vi "ROI-databuffer.vi"(4 "array in":cluster{"x":sgl, "y":sgl}[](array[cluster]), 5 "command":enum16{"get", "set", "clear", "append"}(ring)) -> (1 "array out":cluster{"x":sgl, "y":sgl}[](array[cluster]))   [LabVIEW 2015]
panel:
  in  "point in":cluster{"x":sgl, "y":sgl}
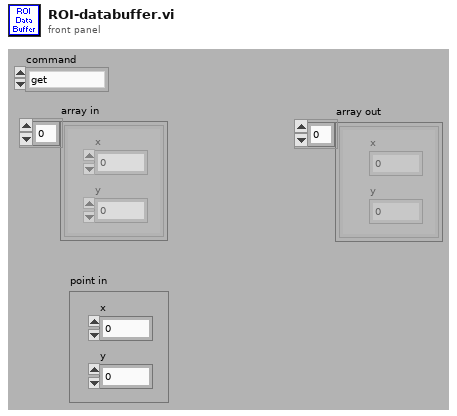
[diagram p1: front panel]
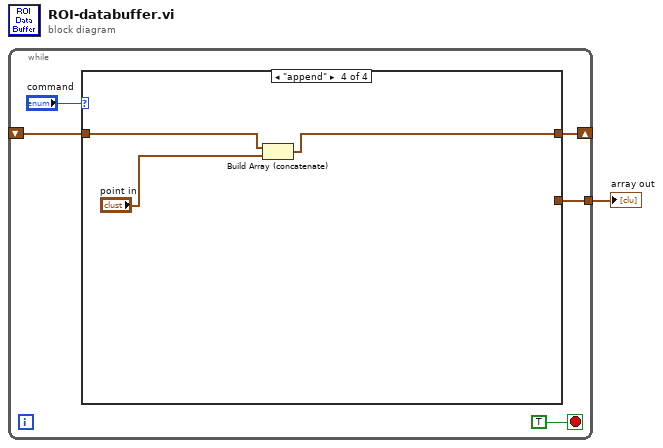
[diagram p0: block diagram]
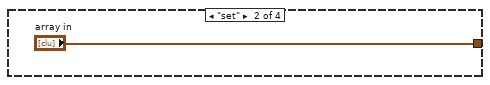
[diagram p3: hidden frame]
diagram:
  n1 = while {
    shift-right: [w4] -> _
    shift-left: _ -> [w5]
    tunnel: [w3] -> w1
    stop <- TRUE stop-if-true
    n2 = case shown="\"append\"" "command" {
      tunnel: [w7 "array in" _ w11] -> w4
      tunnel: w5 -> [w7 _ _ w10]
      tunnel: [w7 _ _ _] -> w3
      frame "get", Default {
      }
      frame "set" {
      }
      frame "clear" {
      }
      frame "append" {
        n3 = Build Array (concatenate)(w10, "point in") -> (w11:cluster{"x":sgl, "y":sgl}[])
      }
    }
  }
  "array out" <- w1
